vi "PropPage_Parallelism.vi"() -> (2 "OKtoQuit":bool)   [LabVIEW 2012]
doc: "Property Page plugin template.\n\n\nGeorge Zou\nhttp://webspace.webring.com/people/og/gtoolbox\n\n2016.7"
uses:
  <resource>/dialog/ParallelSchedulesRadioControl.ctl
  <vilib>/PropPageSupport/pp_TabRef.ctl
  <vilib>/Utility/miscctls.llb/LVParallelSchedulesEnum.ctl
panel:
  in  "TabRef":T1
  in  "QueueName":string
  in  "Main Ref Array In":refnum<vi>[](array[refnum])
  in  "TabCaption":string="Parallelism" caption="Tab Caption"
  in  "id":i32=1 caption="Page ID"
  in  "debug":bool caption="Allow debugging\n(Forces iterations to execute sequentially)"
  in  "partitioning":T2 caption="Iteration partitioning among instances"
  in  "instances":i32 caption="Number of generated parallel loop instances"
  in  "parallelism":bool caption="Enable loop iteration parallelism"
  in  "close":bool caption="Close"
  # "Do not change.  Input/output used by the caller.\nTake a look PropPage_TabularAppearance.vi.  Max FP to see input/output."
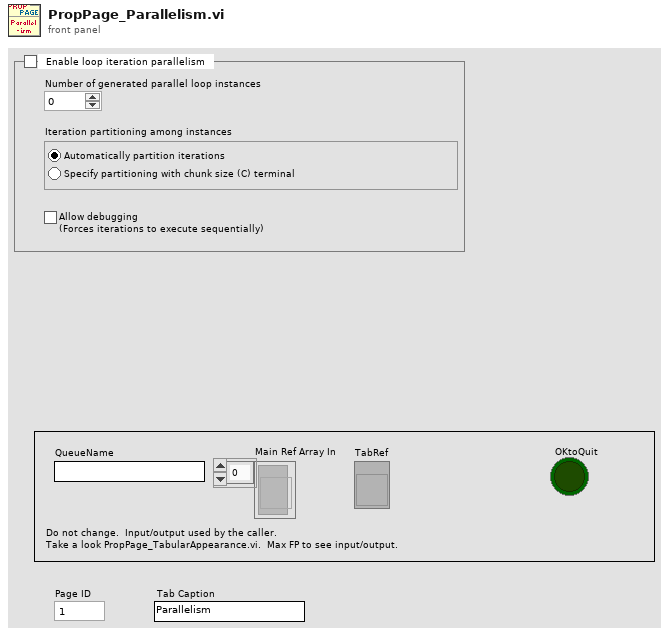
[diagram p1: front panel]
types:
  T1 = typedef "pp_TabRef.ctl" = refnum<vi>
  T2 = typedef "ParallelSchedulesRadioControl.ctl" = enum32{"Automatically partition iterations", "Specify partitioning with chunk size (C) terminal"}
  T3 = enum8{"Enabled", "Disabled", "Disabled and Grayed Out"}
  T4 = typedef "LVParallelSchedulesEnum.ctl" = enum8{"Dynamic decreasing", "Dynamic fixed size", "Static block", "Static block-cyclic"}
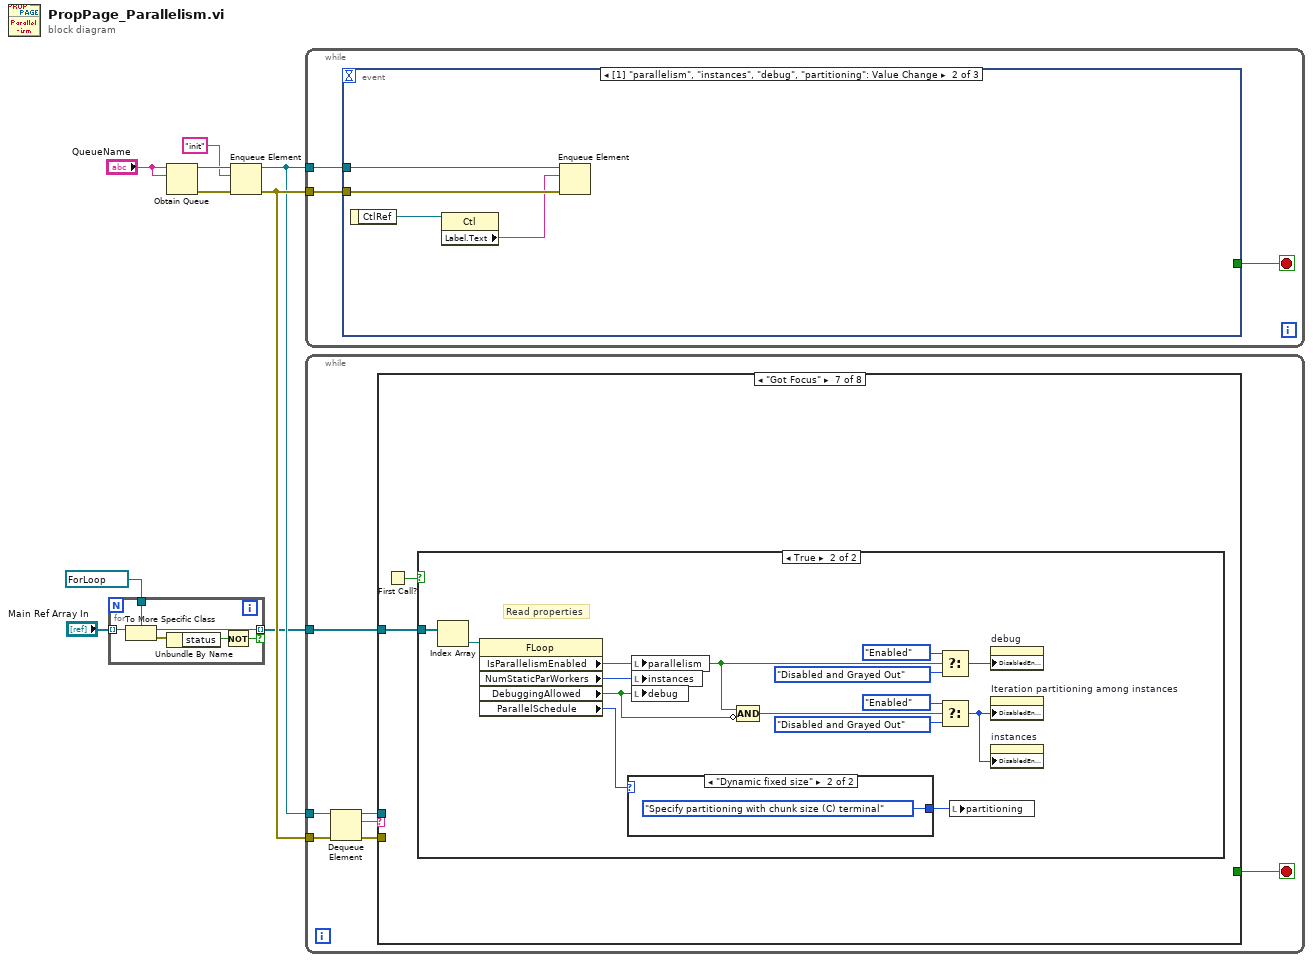
[diagram p0: block diagram]
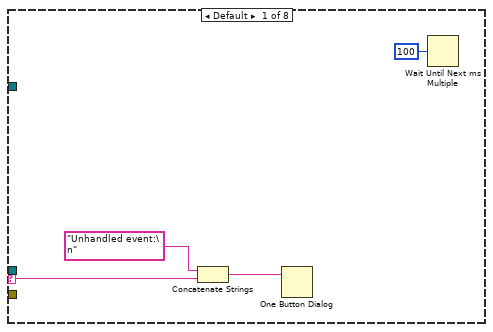
[diagram p2: hidden frame]
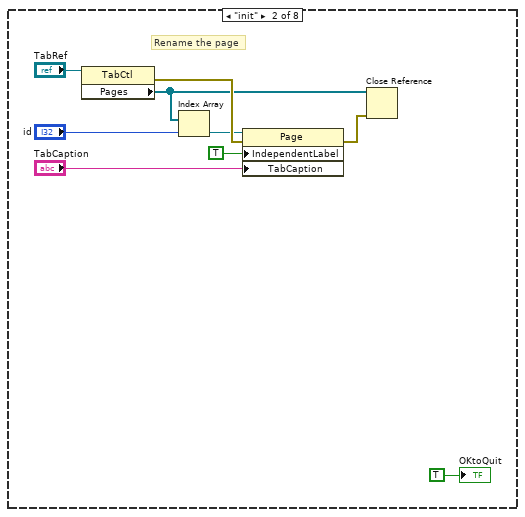
[diagram p3: hidden frame]
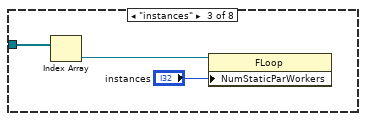
[diagram p4: hidden frame]
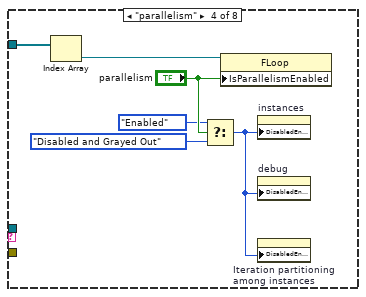
[diagram p5: hidden frame]
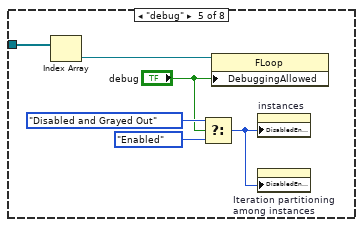
[diagram p6: hidden frame]
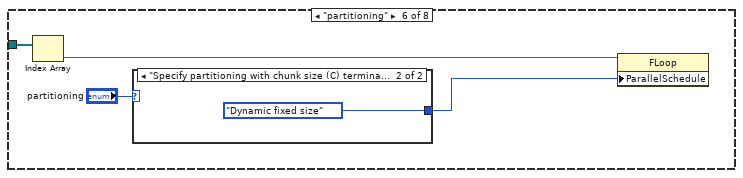
[diagram p7: hidden frame]
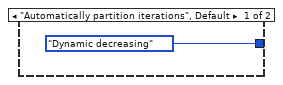
[diagram p8: hidden frame]
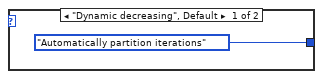
[diagram p10: hidden frame]
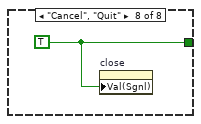
[diagram p11: hidden frame]
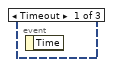
[diagram p12: hidden frame]
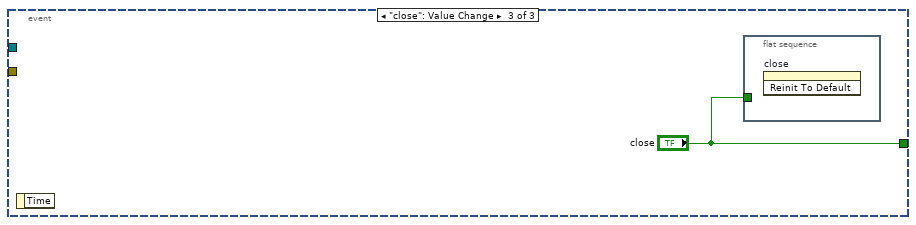
[diagram p13: hidden frame]
diagram:
  n1 = for {
    tunnel: "Main Ref Array In" -> [w15] mode=indexing
    tunnel: refnum<vi> refnum ("FLoop Refnum") -> [w14]
    tunnel: [w13] -> w1 mode=indexing if=w10
    n2 = To More Specific Class(target class=w14, reference=w15) -> (specific class reference=w13:refnum<vi>, error out=w12:errorcluster)  [unwired: 1 in]
    n3 = Unbundle By Name(w12) -> ("status"=w11:bool)
    n4 = Not(x=w11) -> (.not. x?=w10:bool)
  }
  n5 = Obtain Queue(name (unnamed)="QueueName", element data type="QueueName") -> (queue out=w6:refnum<queue>, error out=w7:errorcluster)  [unwired: 3 in, 1 out]
  n6 = Enqueue Element(queue=w6, element="init" ("event"), error in (no error)=w7) -> (queue out=w8:refnum<queue>, error out=w9:errorcluster)  [unwired: 1 in, 1 out]
  n7 = while {
    tunnel: w8 -> [w18]
    tunnel: w9 -> [w17]
    stop <- w16 stop-if-true
    n8 = event shown="[1] \"parallelism\", \"instances\", \"debug\", \"partitioning\": Value Change" {
      selector: _ -> [_ _ _]
      dyn-events: _ -> [_ _ _]
      timeout: _ -> [_ _ _]
      tunnel: w18 -> [_ w22 _]
      tunnel: w17 -> [_ w21 _]
      tunnel: [_ _ "close"] -> w16
      event Timeout {
        n9 = event-data() -> ()  [unwired: 1 in, 1 out]
      }
      event "parallelism", "instances", "debug": Value Change {
        n10 = event-data() -> ("CtlRef"=w20:refnum<vi>)  [unwired: 1 in]
        n11 = property class="Ctl"(reference=w20) -> ("Label.Text"=w19:string)  [unwired: 1 in, 2 out]
        n12 = Enqueue Element(queue=w22, element=w19, error in (no error)=w21) -> ()  [unwired: 1 in, 3 out]
      }
      event "close": Value Change {
        n13 = event-data() -> ()  [unwired: 1 in, 1 out]
        n14 = flat-sequence {
          tunnel: "close" -> [_]
          frame #0 {
            n15 = invoke on="close" class="Bool (strict)" method="Reinit To Default"() -> ()  [unwired: 3 in, 3 out]
          }
        }
      }
    }
  }
  n16 = while {
    tunnel: w9 -> [w30]
    tunnel: w8 -> [w29]
    tunnel: w1 -> [w25]
    stop <- w27 stop-if-true
    n17 = Dequeue Element(queue=w29, error in (no error)=w30) -> (queue out=w26:refnum<queue>, element=w24:string, error out=w28:errorcluster)  [unwired: 1 in, 1 out]
    n18 = case shown="\"Got Focus\"" w24 {
      selector: w24 -> [w34 _ _ _ _ _ _ _]
      tunnel: w28 -> [_ _ _ _ _ _ _ _]
      tunnel: [_ _ _ _ _ _ _ w83] -> w27
      tunnel: w26 -> [_ _ _ _ _ _ _ _]
      tunnel: w25 -> [_ _ w45 w52 w57 w61 w65 _]
      frame Default {
        n19 = Concatenate Strings("Unhandled event:\n" ("string"), w34) -> (w33:string)
        n20 = One Button Dialog(message=w33) -> ()  [unwired: 1 in, 1 out]
        n21 = Wait Until Next ms Multiple(millisecond multiple=u32 100) -> ()  [unwired: 1 out]
      }
      frame "init" {
        # "Rename the page"
        n22 = property class="TabCtl"(reference="TabRef") -> (error out=w43:errorcluster, "Pages"=w35:refnum<vi>[])  [unwired: 1 in, 1 out]
        n23 = Index Array(array=w35, index="id") -> (element=w39:refnum<vi>)
        n24 = property class="Page"(reference=w39, error in=w43, "IndependentLabel"=TRUE ("Independent Label"), "TabCaption"="TabCaption") -> (error out=w36:errorcluster)  [unwired: 1 out]
        n25 = Close Reference(reference=w35, error in (no error)=w36) -> ()  [unwired: 1 out]
        "OKtoQuit" <- TRUE ("OKtoQuit")
      }
      frame "instances" {
        n26 = Index Array(array=w45) -> (element=w46:refnum<vi>)  [unwired: 1 in]
        n27 = property class="FLoop"(reference=w46, "NumStaticParWorkers"="instances") -> ()  [unwired: 1 in, 2 out]
      }
      frame "parallelism" {
        n28 = Index Array(array=w52) -> (element=w51:refnum<vi>)  [unwired: 1 in]
        n29 = Select(t=T3."Enabled" ("Disabled"), s="parallelism", f=T3."Disabled and Grayed Out" ("Disabled")) -> (s? t:f=w47:T3)
        n30 = property class="FLoop"(reference=w51, "IsParallelismEnabled"="parallelism") -> ()  [unwired: 1 in, 2 out]
        n31 = property on="instances" class="DigNum (strict)"("DisabledEnum"=w47) -> ()  [unwired: 2 in, 2 out]
        n32 = property on="debug" class="Bool (strict)"("DisabledEnum"=w47) -> ()  [unwired: 2 in, 2 out]
        n33 = property on="Iteration partitioning among instances" class="RadioBtnsControl (strict)"("DisabledEnum"=w47) -> ()  [unwired: 2 in, 2 out]
      }
      frame "debug" {
        n34 = Index Array(array=w57) -> (element=w58:refnum<vi>)  [unwired: 1 in]
        n35 = Select(t=T3."Disabled and Grayed Out" ("Disabled"), s="debug", f=T3."Enabled" ("Disabled")) -> (s? t:f=w53:T3)
        n36 = property class="FLoop"(reference=w58, "DebuggingAllowed"="debug") -> ()  [unwired: 1 in, 2 out]
        n37 = property on="instances" class="DigNum (strict)"("DisabledEnum"=w53) -> ()  [unwired: 2 in, 2 out]
        n38 = property on="Iteration partitioning among instances" class="RadioBtnsControl (strict)"("DisabledEnum"=w53) -> ()  [unwired: 2 in, 2 out]
      }
      frame "partitioning" {
        n39 = Index Array(array=w61) -> (element=w62:refnum<vi>)  [unwired: 1 in]
        n40 = case shown="\"Specify partitioning with chunk size (C) terminal\"" "partitioning" {
          tunnel: [LVParallelSchedulesEnum."Dynamic decreasing" ("Parallel Schedule") LVParallelSchedulesEnum."Dynamic fixed size" ("Parallel Schedule")] -> w59
          frame "Automatically partition iterations", Default {
          }
          frame "Specify partitioning with chunk size (C) terminal" {
          }
        }
        n41 = property class="FLoop"(reference=w62, "ParallelSchedule"=w59) -> ()  [unwired: 1 in, 2 out]
      }
      frame "Got Focus" {
        n42 = First Call?() -> (First Call?: T/F=w66:bool)
        n43 = case shown="True" w66 {
          tunnel: w65 -> [_ w67]
          frame False {
          }
          frame True {
            # "Read properties"
            n44 = Index Array(array=w67) -> (element=w80:refnum<vi>)  [unwired: 1 in]
            n45 = property class="FLoop"(reference=w80) -> ("IsParallelismEnabled"=w73:bool, "NumStaticParWorkers"=w79:i32, "DebuggingAllowed"=w72:bool, "ParallelSchedule"=w76:T4)  [unwired: 1 in, 2 out]
            n46 = case shown="\"Dynamic fixed size\"" w76 {
              tunnel: [ParallelSchedulesRadioControl."Automatically partition iterations" ("Iteration partitioning among instances") ParallelSchedulesRadioControl."Specify partitioning with chunk size (C) terminal" ("Iteration partitioning among instances")] -> w75
              frame "Dynamic decreasing", Default {
              }
              frame "Dynamic fixed size" {
              }
            }
            n47 = local write "parallelism"(w73) -> ()
            n48 = local write "instances"(w79) -> ()
            n49 = local write "debug"(w72) -> ()
            n50 = Compound Arithmetic op=AND(w73, invert w72) -> (w71:bool)
            n51 = Select(t=T3."Enabled" ("Disabled"), s=w73, f=T3."Disabled and Grayed Out" ("Disabled")) -> (s? t:f=w74:T3)
            n52 = Select(t=T3."Enabled" ("Disabled"), s=w71, f=T3."Disabled and Grayed Out" ("Disabled")) -> (s? t:f=w68:T3)
            n53 = local write "partitioning"(w75) -> ()
            n54 = property on="debug" class="Bool (strict)"("DisabledEnum"=w74) -> ()  [unwired: 2 in, 2 out]
            n55 = property on="Iteration partitioning among instances" class="RadioBtnsControl (strict)"("DisabledEnum"=w68) -> ()  [unwired: 2 in, 2 out]
            n56 = property on="instances" class="DigNum (strict)"("DisabledEnum"=w68) -> ()  [unwired: 2 in, 2 out]
          }
        }
      }
      frame "Cancel", "Quit" {
        w83 = TRUE
        n57 = property on="close" class="Bool (strict)"("Val(Sgnl)"=w83) -> ()  [unwired: 2 in, 2 out]
      }
    }
  }
